vi "path_point_generator.vi"(8 "wheel angle":i8, 11 "distance":u16) -> (0 "y position":i16, 3 "x position":i16)   [LabVIEW 2009]
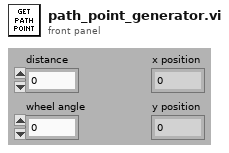
[diagram p1: front panel]
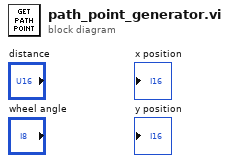
[diagram p0: block diagram]
diagram:
